vi "DIO Pin To Channel.vi"(8 "Error In":errorcluster, 10 "DIO Pins":u8[](array[numeric])) -> (0 "Error Out":errorcluster, 2 "DIO Channels":string[](array[string]))   [LabVIEW 2013]
uses:
  <vilib>/LabVIEW Hacker/LINX/Private/myRIO/myRIO.lvlib
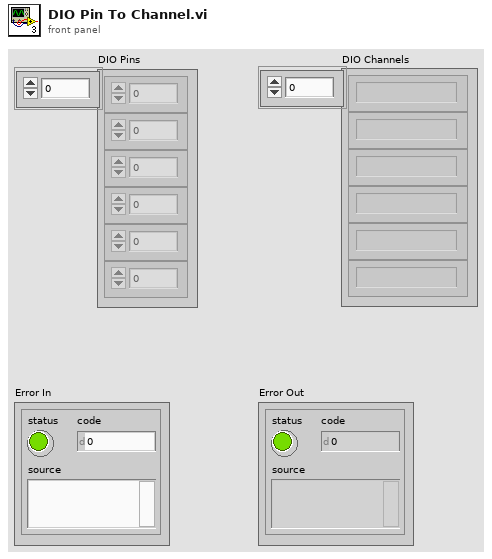
[diagram p1: front panel]
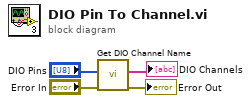
[diagram p0: block diagram]
diagram:
  n1 = call <vilib>:"Get DIO Channel Name.vi"("Error In"="Error In", "DIO Channel Nums"="DIO Pins") -> ("Error Out"=→"Error Out":errorcluster, "DIO Channels"=→"DIO Channels":string[])  [unwired: 8 in]
